vi "dfd_Compute Aliasing Distortion of Filter Banks.vi"(7 "# freq bins":i32=512, 8 "error in (no error)":errorcluster, 9 "dB on? (T)":bool=TRUE, 10 "synthesis bank":T1 {"mBank_Type" items=["Uniform", "Non-Uniform"]; "mBank_Filters"."mMRate_SumWl" min=1 max=32 step=1; "mBank_Filters"."mMRate_InputIwl" min=1 max=32 step=1; "mBank_Filters"."mMRate_GainWl" min=1 max=32 step=1; "mBank_Filters"."mMRate_OutputWl" min=1 max=32 step=1; "mBank_Filters"."mMRate_InputWl" min=1 max=32 step=1; "mBank_Filters"."mMRate_CoefWl" min=1 max=32 step=1; "mBank_Filters"."mMRate_Mode" items=["Default"=-1, "No Rate Change"=0, "Interpolation"=1, "Decimation"=2, "Interpolated"=3, "Rational"=4]}, 11 "analysis bank":T1 {"mBank_Type" items=["Uniform", "Non-Uniform"]; "mBank_Filters"."mMRate_SumWl" min=1 max=32 step=1; "mBank_Filters"."mMRate_InputIwl" min=1 max=32 step=1; "mBank_Filters"."mMRate_GainWl" min=1 max=32 step=1; "mBank_Filters"."mMRate_OutputWl" min=1 max=32 step=1; "mBank_Filters"."mMRate_InputWl" min=1 max=32 step=1; "mBank_Filters"."mMRate_CoefWl" min=1 max=32 step=1; "mBank_Filters"."mMRate_Mode" items=["Default"=-1, "No Rate Change"=0, "Interpolation"=1, "Decimation"=2, "Interpolated"=3, "Rational"=4]}) -> (0 "error out":errorcluster, 3 "aliasing distortion":dbl[](array[numeric]))   [LabVIEW 2017, in "NI_DigFilter_FilterBank.lvlib"]
uses:
  <vilib>/addons/Digital Filter Design/NI_DigFilter_FilterBank.lvlib
  <vilib>/addons/Digital Filter Design/FilterBank.llb/Object/DFD Bank Obj.ctl
  <vilib>/addons/Digital Filter Design/_Objects.llb/DFD Multirate Filter Obj.ctl
  <vilib>/addons/Digital Filter Design/_Objects.llb/DFD Multirate Mode.ctl
  <vilib>/addons/Digital Filter Design/_Objects.llb/DFD Coef Norm Type.ctl
  <vilib>/addons/Digital Filter Design/_Objects.llb/DFD Round-off Mode.ctl
  <vilib>/addons/Digital Filter Design/_Objects.llb/DFD FXP MRate Multiply Mode.ctl
  <vilib>/addons/Digital Filter Design/FilterBank.llb/Object/DFD Filter Bank Processing Method.ctl
  <vilib>/addons/Digital Filter Design/FilterBank.llb/Object/DFD Filter Bank Type.ctl
  <vilib>/addons/Digital Filter Design/NI_DigFilterLicensed.lvlib
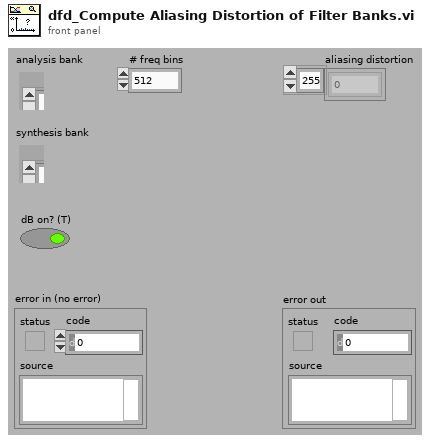
[diagram p1: front panel]
types:
  T1 = typedef "NI_DigFilter_FilterBank.lvlib/DFD Bank Obj.ctl" = cluster{"mBank_Filters":T2[], " mBank_#Bands":i32, "mBank_ProcMethod":T7, "mBank_Coeffs":dbl[], "mBank_Gain":dbl, "mBank_Type":T8}
  T2 = typedef "NI_DigFilterLicensed.lvlib/DFD Multirate Filter Obj.ctl" = cluster{"mMRate_Structure":enum16{"CIC", "FIR", "IIR", "Lattice"}, "mMRate_Mode":T3, "mMRate_Factor":i32, "mMRate_FIRParams":cluster{"mMRate_FIR_H":dbl[], "mMRate_FIR_IsNyquist?":bool, "mMRate_FIR_IsSymmetric?":bool}, "mMRate_CICParams":cluster{"mMRate_CIC_#Stage":i32, "mMRate_CIC_Lag":i32, "mMRate_CIC_Type":enum16{"Lowpass", "Highpass"}}, "mMRate_Order":i32, "mMRate_Version":string, "mMRate_Comments":string, "mMRate_RationalFactor":cluster{"mMRate_L":i32, "mMRate_M":i32}, "mMRate_Fs":dbl, "mMRate_Quantized?":bool, "mMRate_QFilterGain":dbl, "mMRate_CoefWl":i16, "mMRate_Scaling":cluster{"mMRate_ScaleByPowerOf2?":bool, "mMRate_ScaleType":T4}, "mMRate_InputWl":i16, "mMRate_OutputWl":i16, "mMRate_OutputMode":T5, "mMRate_MultMode":T6, "mMRate_BitPruning":bool, "mMRate_GainWl":i16, "mMRate_OutputFwl":i16, "mMRate_SumIwl":i16, "mMRate_InputIwl ":i16, "mMRate_SumWl":i16, "mMRate_CoefIwl":i16}
  T3 = typedef "NI_DigFilterLicensed.lvlib/DFD Multirate Mode.ctl" = i16
  T4 = typedef "NI_DigFilterLicensed.lvlib/DFD Coef Norm Type.ctl" = enum16{"No Norm", "Time Domain 1-Norm", "Time Domain 2-Norm", "Time Domain Inf-Norm"}
  T5 = typedef "NI_DigFilterLicensed.lvlib/DFD Round-off Mode.ctl" = enum16{"Nearest", "Truncation"}
  T6 = typedef "NI_DigFilterLicensed.lvlib/DFD FXP MRate Multiply Mode.ctl" = enum16{"Truncated", "Full"}
  T7 = typedef "NI_DigFilter_FilterBank.lvlib/DFD Filter Bank Processing Method.ctl" = enum16{"General", "2-Band QMF Lattice", "Cosine-Modulated"}
  T8 = typedef "NI_DigFilter_FilterBank.lvlib/DFD Filter Bank Type.ctl" = u16
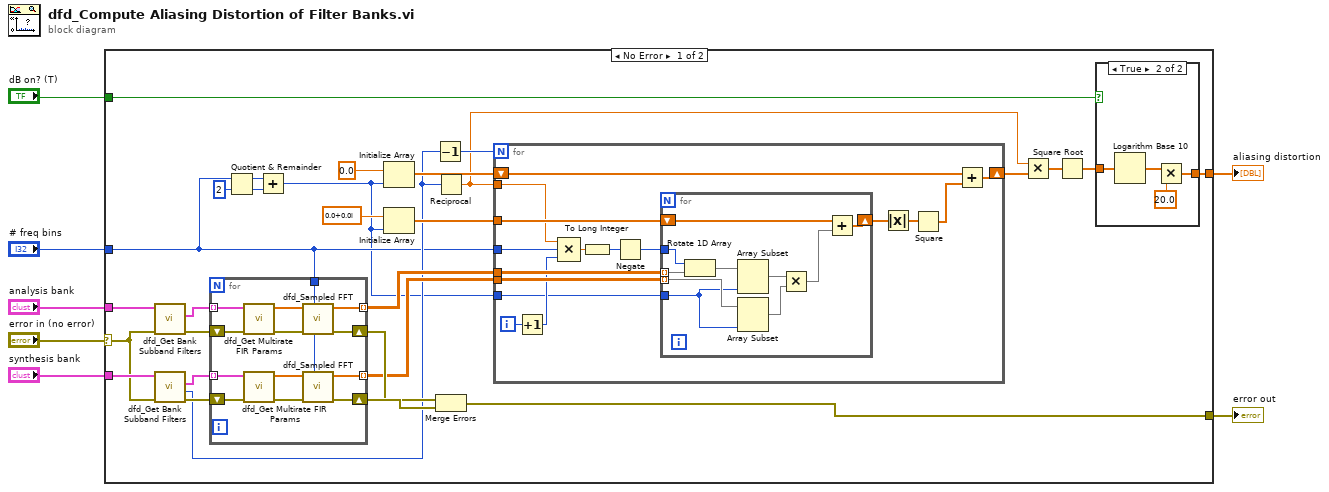
[diagram p0: block diagram]
diagram:
  n1 = case shown="No Error" "error in (no error)" {
    selector: "error in (no error)" -> [w24 w79]
    tunnel: "analysis bank" -> [w35 _]
    tunnel: "synthesis bank" -> [w34 _]
    tunnel: "dB on? (T)" -> [w33 _]
    tunnel: [w32 _] -> w4
    tunnel: "# freq bins" -> [w16 _]
    tunnel: [w23 w79] -> w1
    frame No Error {
      n2 = call <vilib>:"dfd_Get Bank Subband Filters.vi"("error in (no error)"=w24, "bank in"=w35) -> ("error out"=w36:errorcluster, "subband filters"=w18:T2[])  [unwired: 6 in, 2 out]
      n3 = call <vilib>:"dfd_Get Bank Subband Filters.vi"("error in (no error)"=w24, "bank in"=w34) -> ("error out"=w27:errorcluster, "number of bands"=w17:i32, "subband filters"=w19:T2[])  [unwired: 6 in, 1 out]
      n4 = for {
        tunnel: w18 -> [w46] mode=indexing
        tunnel: [w48] -> w22 mode=indexing
        tunnel: w19 -> [w52] mode=indexing
        tunnel: [w49] -> w21 mode=indexing
        tunnel: w16 -> [w42]
        shift-right: [w51] -> w25
        shift-left: w36 -> [w45]
        shift-right: [w43] -> w26
        shift-left: w27 -> [w44]
        n5 = call <vilib>:"dfd_Get Multirate FIR Params.vi"("error in (no error)"=w45, "multirate filter in"=w46) -> ("error out"=w51:errorcluster, "h (n)"=w47:dbl[])  [unwired: 5 in, 3 out]
        n6 = call <vilib>:"dfd_Get Multirate FIR Params.vi"("error in (no error)"=w44, "multirate filter in"=w52) -> ("error out"=w43:errorcluster, "h (n)"=w50:dbl[])  [unwired: 5 in, 3 out]
        n7 = call <vilib>:"dfd_Sampled FFT.vi"("# freq bins (512)"=w42, "h[n]"=w47) -> ("FFT {X}"=w48:cdb[])  [unwired: 9 in]
        n8 = call <vilib>:"dfd_Sampled FFT.vi"("# freq bins (512)"=w42, "h[n]"=w50) -> ("FFT {X}"=w49:cdb[])  [unwired: 9 in]
      }
      n9 = Quotient & Remainder(x=w16, y=2 ("floor(x/y)")) -> (x-y*floor(x/y)=w12:i32, floor(x/y)=w14:i32)
      n10 = Add(x=w12, y=w14) -> (x+y=w13:i32)
      n11 = Initialize Array(0.0, w13) -> (w31:dbl[])
      n12 = Initialize Array(cdb 0.0+0.0i, w13) -> (w29:cdb[])
      n13 = Decrement(x=w17) -> (x-1=w20:i32)
      n14 = Reciprocal(x=w17) -> (1/x=w9:dbl)
      n15 = Merge Errors(w25, w26) -> (w23:errorcluster)
      n16 = for {
        N: w20 -> [_]
        tunnel: w21 -> [w67]
        tunnel: w22 -> [w68]
        tunnel: w29 -> [w66]
        tunnel: w16 -> [w60]
        shift-right: [w63] -> w10
        shift-left: w31 -> [w64]
        tunnel: w9 -> [w57]
        tunnel: w13 -> [w55]
        i -> [w65]
        n17 = Increment(x=w65) -> (x+1=w58:i32)
        n18 = Compound Arithmetic op=MULTIPLY(w57, w60, w58) -> (w62:dbl)
        n19 = To Long Integer(number=w62) -> (32bit integer=w61:i32)
        n20 = Negate(x=w61) -> (-x=w59:i32)
        n21 = for {
          tunnel: w67 -> [w73] mode=indexing
          tunnel: w68 -> [w76] mode=indexing
          shift-right: [w77] -> w54
          shift-left: w66 -> [w78]
          tunnel: w59 -> [w75]
          tunnel: w55 -> [w72]
          n22 = Rotate 1D Array(1:w76, 2:w75) -> (0:w74:cdb[])
          n23 = Array Subset(array=w74, length=w72) -> (w71:cdb[])  [unwired: 1 in]
          n24 = Array Subset(array=w73, length=w72) -> (w70:cdb[])  [unwired: 1 in]
          n25 = Multiply(x=w71, y=w70) -> (x*y=w69:cdb[])
          n26 = Add(x=w78, y=w69) -> (x+y=w77:cdb[])
        }
        n27 = Absolute Value(x=w54) -> (abs(x)=w53:dbl[])
        n28 = Square(x=w53) -> (x^2=w56:dbl[])
        n29 = Add(x=w64, y=w56) -> (x+y=w63:dbl[])
      }
      n30 = Multiply(x=w9, y=w10) -> (x*y=w8:dbl[])
      n31 = Square Root(x=w8) -> (sqrt(x)=w11:dbl[])
      n32 = case shown="True" w33 {
        tunnel: w11 -> [w37 w41]
        tunnel: [w37 w39] -> w32
        frame False {
        }
        frame True {
          n33 = Logarithm Base 10(1:w41) -> (0:w40:dbl[])
          n34 = Multiply(x=w40, y=20.0) -> (x*y=w39:dbl[])
        }
      }
    }
    frame Error {
    }
  }
  "aliasing distortion" <- w4
  "error out" <- w1
